vi "dsdll_stability_demo.vi"() -> ()   [LabVIEW 2020, in "dsdll.lvlib"]
doc: "Simple DSDLL demo for testing the stability of the phase and amplitude.\n\nThe VI generates a sine wave loop at the output. The sine wave frequency is always rounded to have 2^N length to ease the processing so it will have never exactly the desired frequency.\nTha capture unit is periodically triggered in given intervals to capture 2^N samples. The waveform is displayed and passed to the FFT to get spectrum of the signal which is also displayed. The DFT bin with the sine wave frequency is selected, phase unrolling based on the first sample time-stamp is applied and the result is displayed.\nIf both wave output and capture sampling are perfectly synchronous and no samples are missing in the captured data the output should be noisy but drift-less phase. In real life there will be always some fluctuations because of temperature dependent components in analog signal path but there should be no continuous drift and especially no jumps."
uses:
  dsdll.lvlib
  dsdll_instance.ctl
  dsdll_device_record.ctl
  dsdll_format.ctl
  dsdll_sample_format.ctl
  dsdll_capture_wave_auto_float32.vi
  dsdll_output_write_auto_float32.vi
panel:
  out "ref phi":dbl caption="Phase [rad]" format="%_7p"
  out "ref time":timestamp
  out "phase [rad]":dbl caption="Phase [rad]" format="%_7p"
  out "magnitude [-]":dbl caption="Magnitude [-]" format="%_6p"
  out "f out [Hz]":dbl=1000.0 caption="Actual f [Hz]"
  in  "f in [Hz]":dbl=1000.0 caption="Genertor f [Hz]"
  out "Stability":cluster{dbl[], dbl[]}[](graph)
  in  "capt n":u16(ring)=32 caption="Capture periods" items=["4"=4, "8"=8, "16"=16, "32"=32, "64"=64, "128"=128]
  in  "srate":u32=48000 caption="Sample rate [Hz]"
  out "Waveforms":cluster{i32[], "float32 waves":sgl[]}(graph)
  out "Spectrum":cluster{dbl[], sgl[]}(graph)
  in  "refresh":i32=250 caption="Refresh [ms]" min=0
  in  "btn clr avg":bool
  in  "btn close":bool
  in  "btn open":bool
  in  "btn exit":bool
  in  "devs capt":u16(ring) caption="Capture devices"
  in  "devs out":u16(ring) caption="Output devices"
  in  "btn enum":bool
  out "error out":errorcluster caption="Error out"
  out "dsdll":T1
  # "DSDLL: Stability demo"
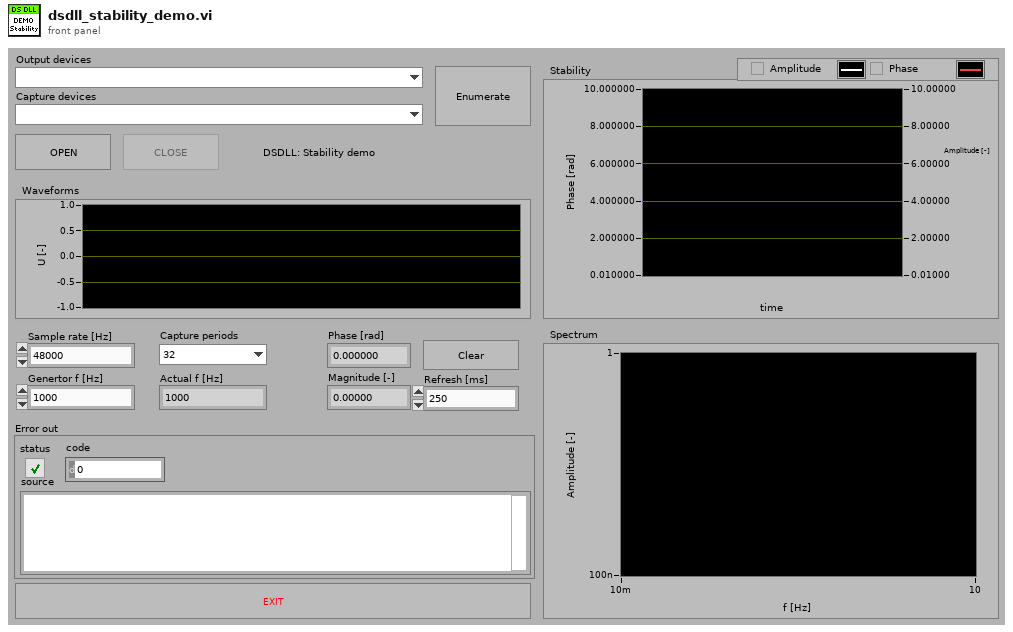
[diagram p1: front panel]
types:
  T1 = typedef "dsdll.lvlib/dsdll_instance.ctl" = cluster{"dsdll path":path, "dsdll handle":u8[], "output devices":T2[], "capture devices":T2[]}
  T2 = typedef "dsdll.lvlib/dsdll_device_record.ctl" = cluster{"guid":u8[], "name":string}
  T3 = typedef "dsdll.lvlib/dsdll_format.ctl" = cluster{"sample rate [Hz]":u32, "out channels":u16, "inp channels":u16, "format":T4}
  T4 = typedef "dsdll.lvlib/dsdll_sample_format.ctl" = enum16{"IEEE float 32", "PCM 16 bit"}
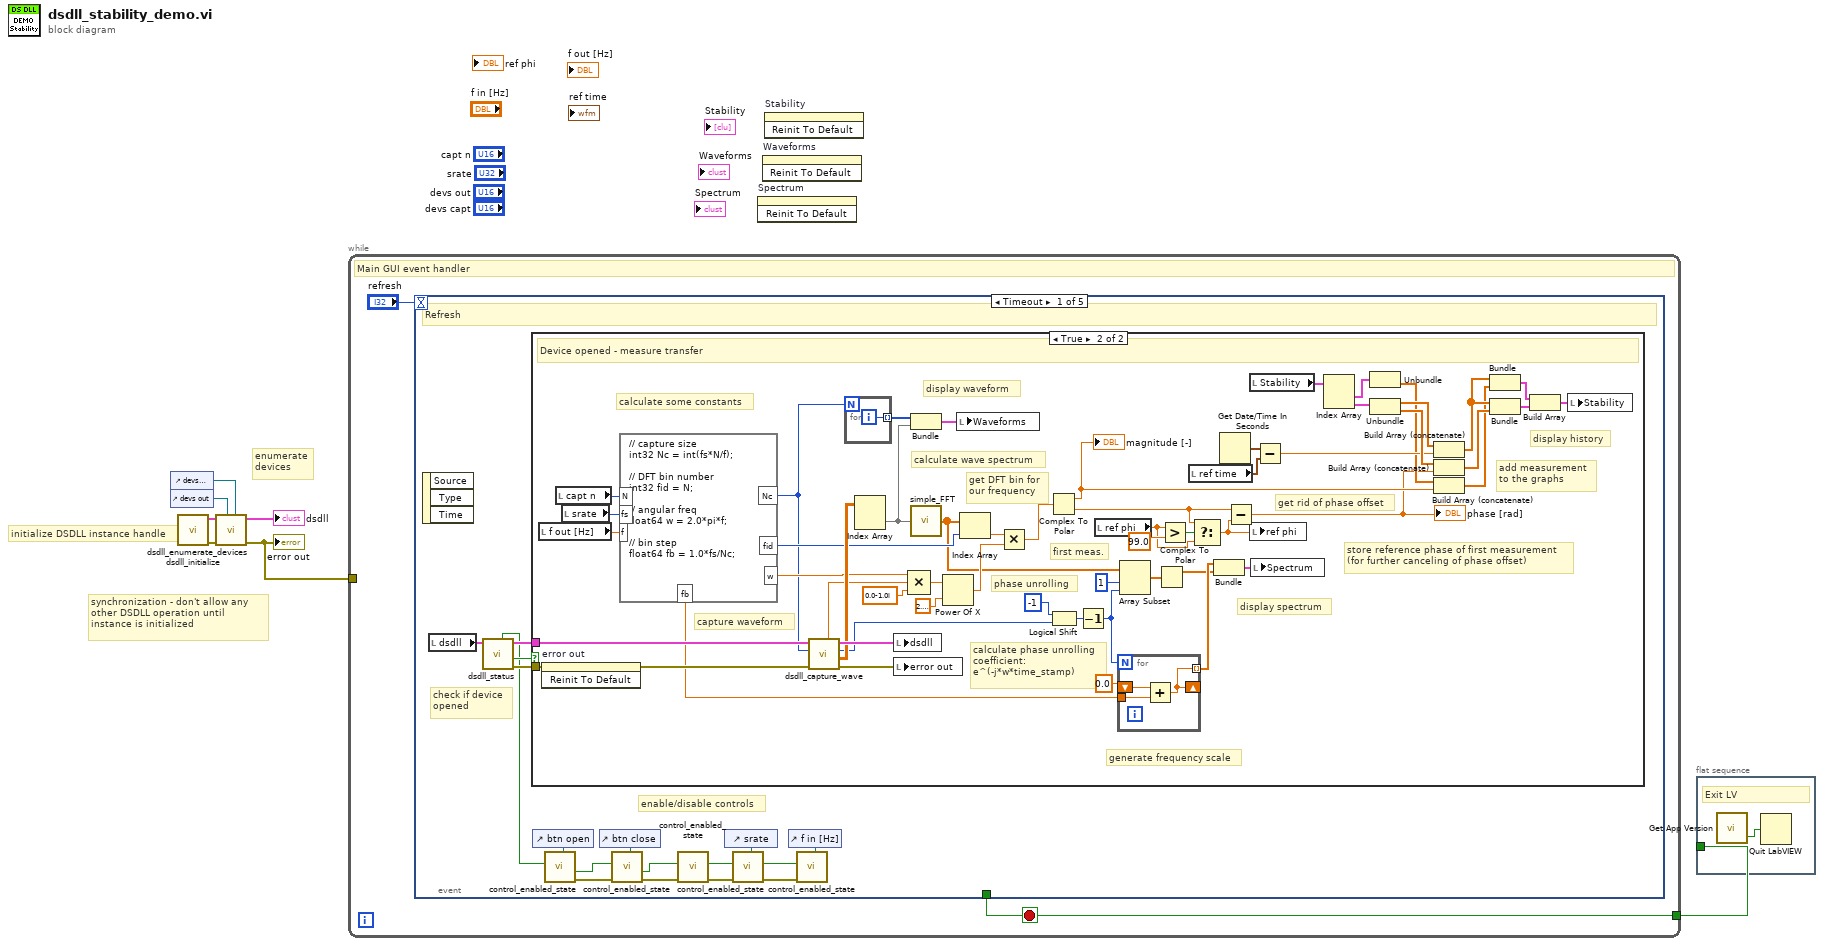
[diagram p0: block diagram]
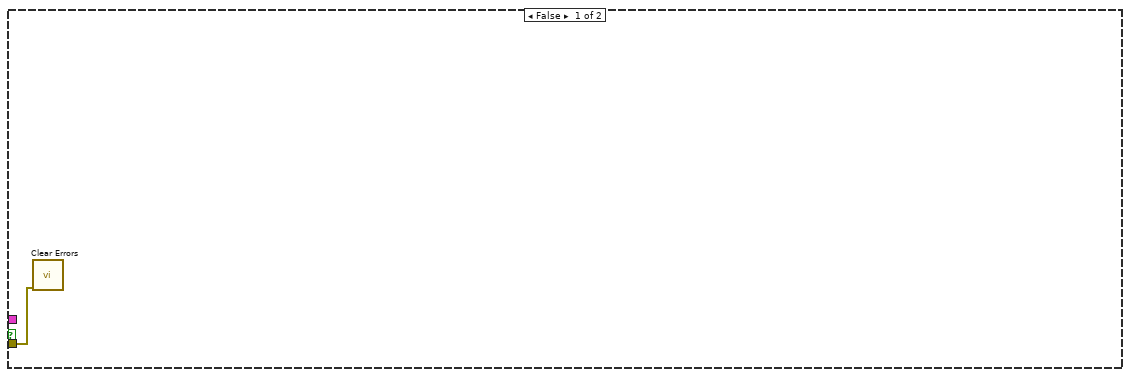
[diagram p2: hidden frame]
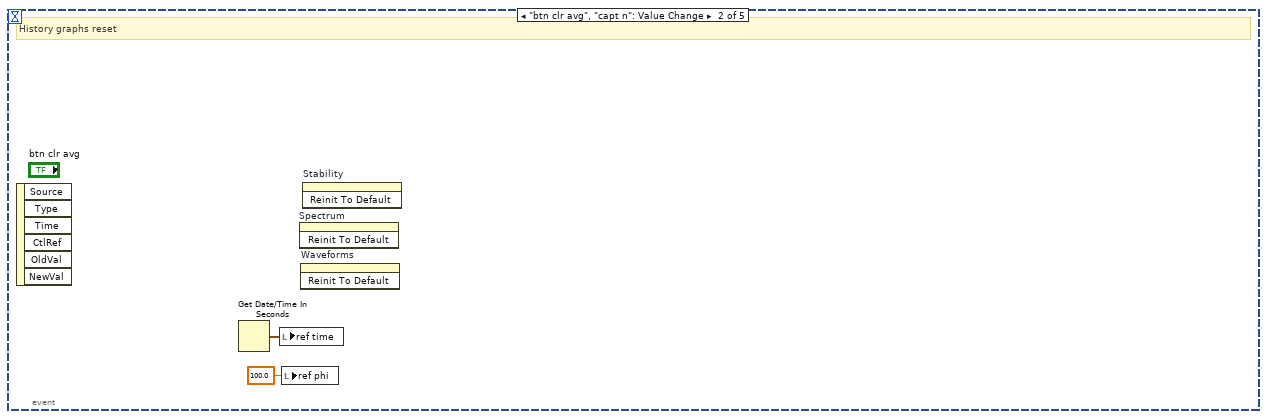
[diagram p3: hidden frame]
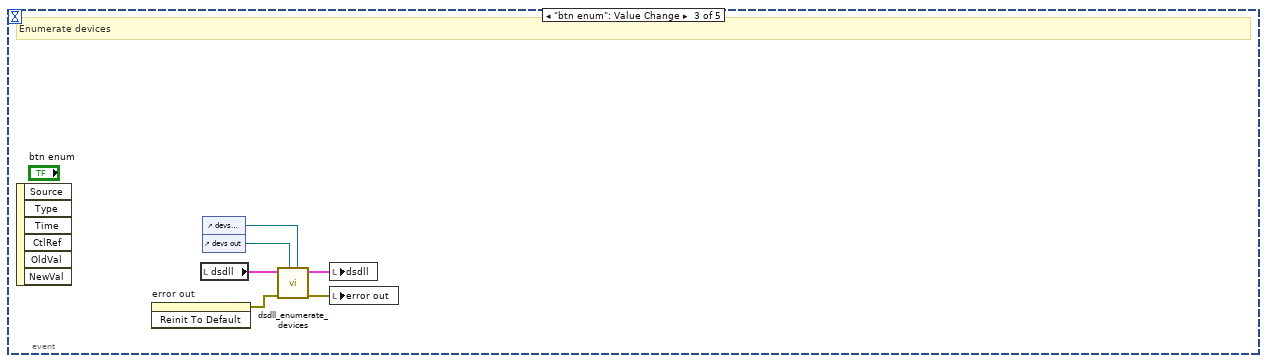
[diagram p4: hidden frame]
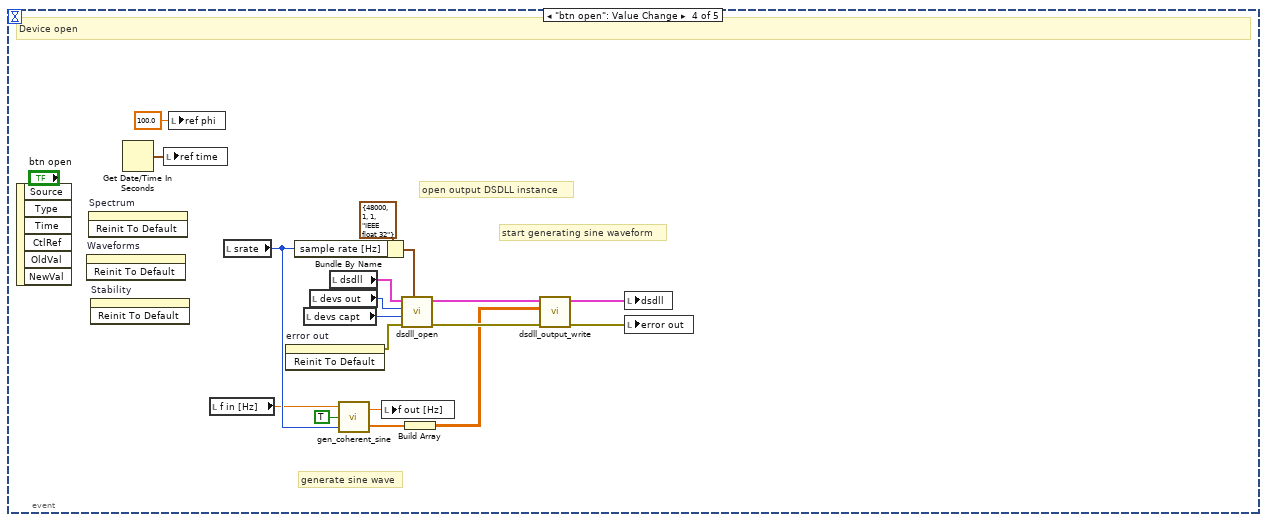
[diagram p5: hidden frame]
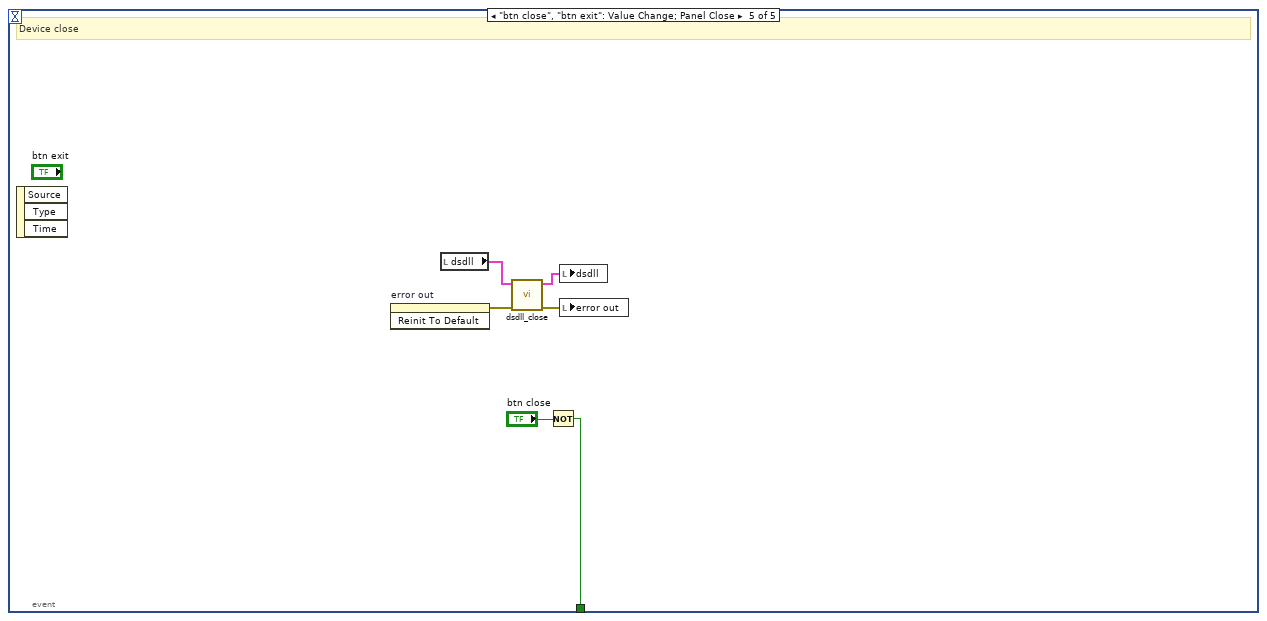
[diagram p6: hidden frame]
diagram:
  # "enumerate\ndevices"
  # "synchronization - don't allow any\nother DSDLL operation until\ninstance is initialized"
  # "initialize DSDLL instance handle"
  n1 = control-ref of="devs capt"() -> (w3:refnum<vi>)
  n2 = control-ref of="devs out"() -> (w4:refnum<vi>)
  n3 = call "dsdll_initialize.vi"() -> ("error out"=w7:errorcluster, "dsdll instance out"=w6:T1)  [unwired: 10 in]
  n4 = call "dsdll_enumerate_devices.vi"("capture devices ring ref"=w3, "output devices ring ref"=w4, "error in"=w7, "dsdll instance in"=w6) -> ("error out"=w1:errorcluster, "dsdll instance out"=→"dsdll":T1)  [unwired: 4 in, 2 out]
  "error out" <- w1
  n5 = while {
    tunnel: [w9] -> w2
    tunnel: w1 -> [_]
    stop <- w9 stop-if-true
    # "Main GUI event handler"
    n6 = event shown="[0] Timeout" {
      selector: _ -> [_ _ _ _ _]
      dyn-events: _ -> [_ _ _ _ _]
      timeout: "refresh" -> [_ _ _ _ _]
      tunnel: [_ _ _ _ w114] -> w9
      event Timeout {
        # "check if device\nopened"
        # "enable/disable controls"
        # "Refresh"
        n7 = event-data() -> ()  [unwired: 1 in, 3 out]
        n8 = local read "dsdll"() -> (w25:T1)
        n9 = call "dsdll_status.vi"("dsdll instance in"=w25) -> ("error out"=w23:errorcluster, "output buffer ok"=w26:bool, "dsdll instance out"=w24:T1, "invalid instance handle"=w20:bool)  [unwired: 5 in, 2 out]
        n10 = case shown="True" w26 {
          tunnel: w24 -> [_ w79]
          tunnel: w23 -> [w27 w77]
          frame False {
            n11 = call <vilib>:"Clear Errors.vi"("error in (no error)"=w27) -> ()  [unwired: 5 in, 2 out]
          }
          frame True {
            # "display history"
            # "add measurement\nto the graphs"
            # "display waveform"
            # "display spectrum"
            # "calculate phase unrolling\ncoefficient:\ne^(-j*w*time_stamp)"
            # "phase unrolling"
            # "calculate some constants"
            # "first meas."
            # "get rid of phase offset"
            # "store reference phase of first measurement\n(for further canceling of phase offset)"
            # "generate frequency scale"
            # "get DFT bin for\nour frequency"
            # "calculate wave spectrum"
            # "capture waveform"
            # "Device opened - measure transfer"
            n12 = local read "f out [Hz]"() -> (w73:dbl)
            n13 = invoke on="error out" class="Clust (strict)" method="Reinit To Default"(error in=w77) -> (error out=w83:errorcluster)  [unwired: 2 in, 2 out]
            n14 = local read "capt n"() -> (w75:u16)
            n15 = local read "srate"() -> (w74:u32)
            n16 = formula code="// capture size\nint32 Nc = int(fs*N/f);\n\n// DFT bin number\nint32 fid = N;\n\n// angular freq\nfloat64 w = 2.0*pi*f;\n\n// bin step\nfloat64 fb = 1.0*fs/Nc;"("N"=w75, "fs"=w74, "f"=w73) -> ("Nc"=w53:i32, "fid"=w72:i32, "w"=w71:dbl, "fb"=w54:dbl)
            n17 = call-poly "dsdll_capture_wave.vi"("error in"=w83, "samples count in"=w53, "dsdll instance in"=w79) -> ("error out"=w82:errorcluster, "float32 waves"=w80:sgl[][], "samples count out"=w52:u32, "dsdll instance out"=w81:T1, "time stamp [s]"=w62:dbl)  [unwired: 3 in, 1 out]
            n18 = for {
              N: w53 -> [_]
              tunnel: [w87] -> w78 mode=indexing
              i -> [w87]
            }
            n19 = Index Array(array=w80) -> (element=w60:sgl[])  [unwired: 2 in]
            n20 = local write "dsdll"(w81) -> ()
            n21 = local write "error out"(w82) -> ()
            n22 = Compound Arithmetic op=MULTIPLY(w71, w62, cdb 0.0-1.0i ("y")) -> (w69:cdb)
            n23 = Bundle(w78, "float32 waves"=w60) -> (w76:cluster{i32[], "float32 waves":sgl[]})  [unwired: 1 in]
            n24 = call "simple_FFT.vi"("x(t)"=w60) -> ("X(w)"=w51:cdb[])
            n25 = Power Of X(1:2.718281828459045, 2:w69) -> (0:w67:cdb)
            n26 = local write "Waveforms"(w76) -> ()
            n27 = Index Array(array=w51, index=w72) -> (element=w68:cdb)
            n28 = Multiply(x=w68, y=w67) -> (x*y=w66:cdb)
            n29 = Complex To Polar(r * e^(i*theta)=w66) -> (r=w34:dbl, theta=w30:dbl)
            "magnitude [-]" <- w34
            n30 = Logical Shift(y=i16 -1, x=w52) -> (x << y=w63:u32)
            n31 = Decrement(x=w63) -> (x-1=w58:u32)
            n32 = local read "ref phi"() -> (w31:dbl)
            n33 = for {
              N: w58 -> [_]
              tunnel: w54 -> [w86]
              shift-right: [w84] -> _
              shift-left: 0.0 -> [w85]
              tunnel: [w84] -> w56 mode=indexing
              n34 = Add(x=w85, y=w86) -> (x+y=w84:dbl)
            }
            n35 = Array Subset(array=w51, index=1, length=w58) -> (w57:cdb[])
            n36 = Complex To Polar(r * e^(i*theta)=w57) -> (r=w55:dbl[])  [unwired: 1 out]
            n37 = Greater?(x=w31, y=99.0) -> (0:w32:bool)
            n38 = local read "ref time"() -> (w45:timestamp)
            n39 = Select(t=w30, s=w32, f=w31) -> (s? t:f=w29:dbl)
            n40 = Bundle(w56, w55) -> (w50:cluster{dbl[], dbl[]})  [unwired: 1 in]
            n41 = Get Date/Time In Seconds() -> (seconds since 1Jan1904=w46:timestamp)
            n42 = Subtract(x=w30, y=w29) -> (x-y=w28:dbl)
            "phase [rad]" <- w28
            n43 = local read "Stability"() -> (w43:cluster{dbl[], dbl[]}[])
            n44 = local write "ref phi"(w29) -> ()
            n45 = local write "Spectrum"(w50) -> ()
            n46 = Subtract(x=w46, y=w45) -> (x-y=w44:dbl)
            n47 = Index Array(array=w43) -> (element #1=w41:cluster{dbl[], dbl[]}, element #2=w42:cluster{dbl[], dbl[]})  [unwired: 2 in]
            n48 = Unbundle(w41) -> (w35:dbl[])  [unwired: 1 out]
            n49 = Unbundle(w42) -> (w49:dbl[], w48:dbl[])
            n50 = Build Array (concatenate)(w49, w44) -> (w38:dbl[])
            n51 = Build Array (concatenate)(w48, w28) -> (w47:dbl[])
            n52 = Build Array (concatenate)(w35, w34) -> (w37:dbl[])
            n53 = Bundle(w38, w37) -> (w39:cluster{dbl[], dbl[]})  [unwired: 1 in]
            n54 = Bundle(w38, w47) -> (w40:cluster{dbl[], dbl[]})  [unwired: 1 in]
            n55 = Build Array(w39, w40) -> (w36:cluster{dbl[], dbl[]}[])
            n56 = local write "Stability"(w36) -> ()
          }
        }
        n57 = control-ref of="btn open"() -> (w22:refnum<vi>)
        n58 = call "control_enabled_state.vi"("enabled"=w20, "control in"=w22) -> ("error out"=w13:errorcluster, "disabled"=w19:bool)  [unwired: 6 in, 2 out]
        n59 = control-ref of="btn close"() -> (w21:refnum<vi>)
        n60 = call "control_enabled_state.vi"("error in (no error)"=w13, "enabled"=w19, "control in"=w21) -> ("error out"=w14:errorcluster, "disabled"=w18:bool)  [unwired: 5 in, 2 out]
        n61 = call "control_enabled_state.vi"("error in (no error)"=w14, "enabled"=w18) -> ("error out"=w16:errorcluster, "enabled"=w15:bool)  [unwired: 6 in, 2 out]
        n62 = control-ref of="srate"() -> (w17:refnum<vi>)
        n63 = call "control_enabled_state.vi"("error in (no error)"=w16, "enabled"=w15, "control in"=w17) -> ("error out"=w10:errorcluster, "enabled"=w11:bool)  [unwired: 5 in, 2 out]
        n64 = control-ref of="f in [Hz]"() -> (w12:refnum<vi>)
        n65 = call "control_enabled_state.vi"("error in (no error)"=w10, "enabled"=w11, "control in"=w12) -> ()  [unwired: 5 in, 4 out]
      }
      event "btn clr avg", "capt n": Value Change {
        # "History graphs reset"
        n66 = event-data() -> ()  [unwired: 1 in, 6 out]
        n67 = Get Date/Time In Seconds() -> (seconds since 1Jan1904=w89:timestamp)
        n68 = local write "ref time"(w89) -> ()
        n69 = local write "ref phi"(100.0 ("ref phi")) -> ()
        n70 = invoke on="Spectrum" class="XYGraph (strict)" method="Reinit To Default"() -> ()  [unwired: 3 in, 3 out]
        n71 = invoke on="Waveforms" class="XYGraph (strict)" method="Reinit To Default"() -> ()  [unwired: 3 in, 3 out]
        n72 = invoke on="Stability" class="XYGraph (strict)" method="Reinit To Default"() -> ()  [unwired: 3 in, 3 out]
      }
      event "btn enum": Value Change {
        # "Enumerate devices"
        n73 = event-data() -> ()  [unwired: 1 in, 6 out]
        n74 = invoke on="error out" class="Clust (strict)" method="Reinit To Default"() -> (error out=w90:errorcluster)  [unwired: 3 in, 2 out]
        n75 = local read "dsdll"() -> (w95:T1)
        n76 = control-ref of="devs capt"() -> (w92:refnum<vi>)
        n77 = control-ref of="devs out"() -> (w93:refnum<vi>)
        n78 = call "dsdll_enumerate_devices.vi"("capture devices ring ref"=w92, "output devices ring ref"=w93, "error in"=w90, "dsdll instance in"=w95) -> ("error out"=w94:errorcluster, "dsdll instance out"=w91:T1)  [unwired: 4 in, 2 out]
        n79 = local write "dsdll"(w91) -> ()
        n80 = local write "error out"(w94) -> ()
      }
      event "btn open": Value Change {
        # "generate sine wave"
        # "start generating sine waveform"
        # "open output DSDLL instance"
        # "Device open"
        n81 = event-data() -> ()  [unwired: 1 in, 6 out]
        n82 = invoke on="Waveforms" class="XYGraph (strict)" method="Reinit To Default"() -> ()  [unwired: 3 in, 3 out]
        n83 = invoke on="Spectrum" class="XYGraph (strict)" method="Reinit To Default"() -> ()  [unwired: 3 in, 3 out]
        n84 = invoke on="Stability" class="XYGraph (strict)" method="Reinit To Default"() -> ()  [unwired: 3 in, 3 out]
        n85 = Get Date/Time In Seconds() -> (seconds since 1Jan1904=w97:timestamp)
        n86 = local write "ref time"(w97) -> ()
        n87 = local write "ref phi"(100.0 ("ref phi")) -> ()
        n88 = local read "f in [Hz]"() -> (w99:dbl)
        n89 = local read "srate"() -> (w102:u32)
        n90 = invoke on="error out" class="Clust (strict)" method="Reinit To Default"() -> (error out=w110:errorcluster)  [unwired: 3 in, 2 out]
        n91 = Bundle By Name(cluster=T3 {"sample rate [Hz]"=48000, "out channels"=1, "inp channels"=1, "format"=enum."IEEE float 32"} ("format"), "sample rate [Hz]"=w102) -> (w103:T3)
        n92 = local read "devs capt"() -> (w112:u16)
        n93 = local read "devs out"() -> (w111:u16)
        n94 = local read "dsdll"() -> (w113:T1)
        n95 = call "gen_coherent_sine.vi"("fs [Hz]"=w102, "limit wave size to power of 2"=TRUE, "f in [Hz]"=w99) -> ("wave"=w101:dbl[], "f out [Hz]"=w100:dbl)
        n96 = local write "f out [Hz]"(w100) -> ()
        n97 = call "dsdll_open.vi"("format"=w103, "error in"=w110, "capture device id"=w112, "output device id"=w111, "dsdll instance in"=w113) -> ("error out"=w109:errorcluster, "dsdll instance out"=w106:T1)  [unwired: 5 in]
        n98 = Build Array(w101) -> (w105:dbl[][])
        n99 = call-poly "dsdll_output_write.vi"("error in"=w109, "float32 samples"=w105, "dsdll instance in"=w106) -> ("error out"=w108:errorcluster, "dsdll instance out"=w107:T1)  [unwired: 7 in]
        n100 = local write "dsdll"(w107) -> ()
        n101 = local write "error out"(w108) -> ()
      }
      event "btn close", "btn exit": Value Change; Panel Close {
        # "Device close"
        n102 = event-data() -> ()  [unwired: 1 in, 3 out]
        n103 = invoke on="error out" class="Clust (strict)" method="Reinit To Default"() -> (error out=w116:errorcluster)  [unwired: 3 in, 2 out]
        n104 = local read "dsdll"() -> (w117:T1)
        n105 = call "dsdll_close.vi"("error in"=w116, "dsdll instance in"=w117) -> ("error out"=w119:errorcluster, "dsdll instance out"=w118:T1)  [unwired: 8 in]
        n106 = Not(x="btn close") -> (.not. x?=w114:bool)
        n107 = local write "dsdll"(w118) -> ()
        n108 = local write "error out"(w119) -> ()
      }
    }
  }
  n109 = invoke on="Spectrum" class="XYGraph (strict)" method="Reinit To Default"() -> ()  [unwired: 3 in, 3 out]
  n110 = invoke on="Waveforms" class="XYGraph (strict)" method="Reinit To Default"() -> ()  [unwired: 3 in, 3 out]
  n111 = invoke on="Stability" class="XYGraph (strict)" method="Reinit To Default"() -> ()  [unwired: 3 in, 3 out]
  n112 = flat-sequence {
    tunnel: w2 -> [_]
    frame #0 {
      # "Exit LV"
      n113 = call "Get App Version.vi"() -> ("runtime"=w120:bool)  [unwired: 1 out]
      n114 = Quit LabVIEW(quit? (T)=w120) -> ()
    }
  }
